vi "ProjectItemRef.vi"(11 "Project Item Refnum":refnum<vi>) -> (2 "Display String":string, 3 "Stop?":bool)   [LabVIEW 2017]
doc: "Displays the project item name, type, path, and hex reference value. You can use this probe to set a breakpoint if the value is an invalid refnum."
uses:
  <vilib>/Utility/error.llb/DialogTypeEnum.ctl
panel:
  in  "ProjItem type":string="Project Item type"
  in  "error source":string="Sring Queue Refnum Probe"
  in  "ProjItem path":string="Project Item path"
  in  "ProjItem name":string="Project Item name"
  in  "Pause if Not a Refnum":bool
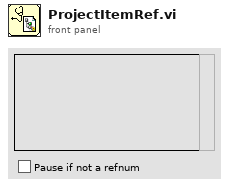
[diagram p1: front panel]
types:
  T1 = typedef "DialogTypeEnum.ctl" = enum16{"no dialog", "OK message", "continue or stop message", "auto error handling dialog", "OK message + warnings", "continue/stop + warnings"}
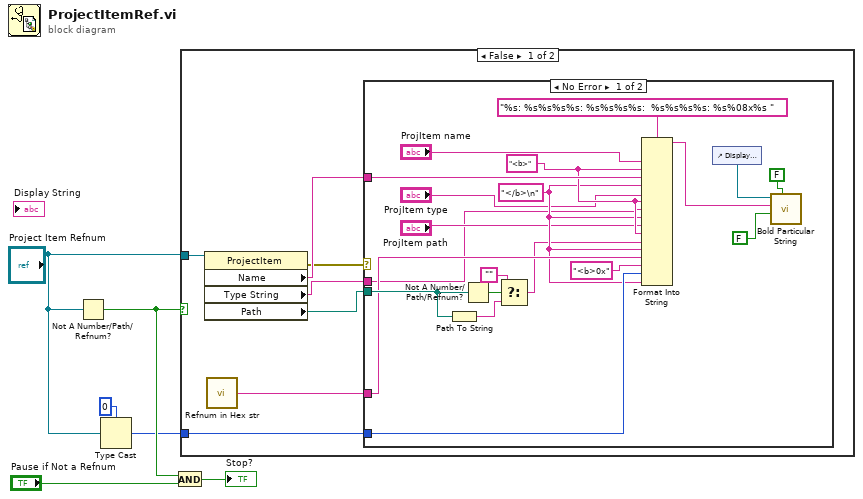
[diagram p0: block diagram]
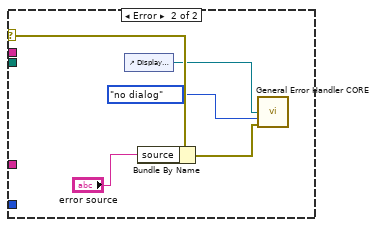
[diagram p2: hidden frame]
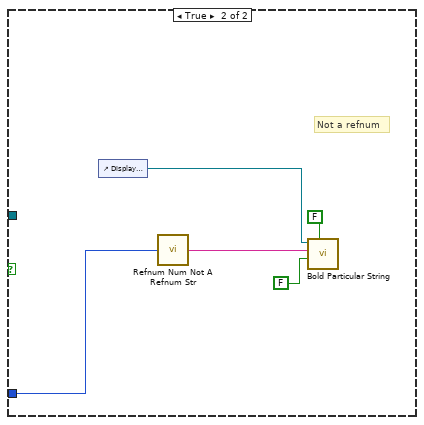
[diagram p3: hidden frame]
diagram:
  n1 = Not A Number/Path/Refnum?(number/path/refnum="Project Item Refnum") -> (NaN/Path/Refnum?=w4:bool)
  n2 = Type Cast(type=u32 0, x="Project Item Refnum") -> (*(type *) &x=w2:u32)
  n3 = And(x=w4, y="Pause if Not a Refnum") -> (x .and. y?=→"Stop?":bool)
  n4 = case shown="False" w4 {
    tunnel: "Project Item Refnum" -> [w11 _]
    tunnel: w2 -> [w12 w39]
    frame False {
      n5 = property class="ProjectItem"(reference=w11) -> (error out=w9:errorcluster, "Name"=w10:string, "Type String"=w7:string, "Path"=w8:path)  [unwired: 1 in, 1 out]
      n6 = call <vilib>:"Refnum in Hex str.vi"() -> ("refnum in hex"=w13:string)
      n7 = case shown="No Error" w9 {
        selector: w9 -> [_ w37]
        tunnel: w10 -> [w32 _]
        tunnel: w12 -> [w19 _]
        tunnel: w13 -> [w21 _]
        tunnel: w8 -> [w23 _]
        tunnel: w7 -> [w15 _]
        frame No Error {
          w18 = "</b>\n"
          w22 = "<b>"
          n8 = Path To String(path=w23) -> (string=w25:string)
          n9 = Not A Number/Path/Refnum?(number/path/refnum=w23) -> (NaN/Path/Refnum?=w26:bool)
          n10 = Select(t="", s=w26, f=w25) -> (s? t:f=w14:string)
          n11 = Format Into String(format string="%s: %s%s%s%s: %s%s%s%s:  %s%s%s%s: %s%08x%s ", "ProjItem name", w22, w32, w18, "ProjItem type", w22, w15, w18, "ProjItem path", w22, w14, w18, w21, "<b>0x", w19, w18) -> (resulting string=w30:string)  [unwired: 2 in, 1 out]
          n12 = control-ref of="Display String"() -> (w31:refnum<vi>)
          n13 = call <vilib>:"Bold Particular String.vi"("Always Refresh? (TRUE)"=FALSE ("Always Refresh? (FALSE)"), "resize string? (TRUE)"=FALSE, "text to display"=w30, "string refnum"=w31) -> ()  [unwired: 6 in, 2 out]
        }
        frame Error {
          n14 = control-ref of="Display String"() -> (w35:refnum<vi>)
          n15 = Bundle By Name(cluster=w37, "source"="error source") -> (w36:errorcluster)
          n16 = call <vilib>:"General Error Handler CORE.vi"("String to Format (not a refnum)"=w35, "type of dialog (OK msg:1)"=DialogTypeEnum."no dialog", "error in (no error)"=w36) -> ()  [unwired: 7 in, 6 out]
        }
      }
    }
    frame True {
      # "Not a refnum"
      n17 = control-ref of="Display String"() -> (w43:refnum<vi>)
      n18 = call <vilib>:"Refnum Num Not A Refnum Str.vi"("Numeric"=w39) -> ("text to display"=w40:string)
      n19 = call <vilib>:"Bold Particular String.vi"("Always Refresh? (TRUE)"=FALSE ("Always Refresh? (FALSE)"), "resize string? (TRUE)"=FALSE, "text to display"=w40, "string refnum"=w43) -> ()  [unwired: 6 in, 2 out]
    }
  }
